vi "runtime execution.vi"() -> (0 "error out":errorcluster)   [LabVIEW 2013, in "shared memory module tests.lvlib"]
uses:
  shared memory module tests.lvlib
  module/execution/shared memory module runtime.lvclass
  module/execution/shared memory module runtime.lvclass/shared memory module runtime.ctl
  <vilib>/NI/Tag Bus/table/data polymorphs/write many/write Doubles.vi
  <vilib>/NI/Tag Bus/table/data polymorphs/write many/write I32s.vi
  <vilib>/NI/Tag Bus/table/data polymorphs/write many/write Booleans.vi
  module/execution/Read inputs.vi
  module/execution/Read outputs.vi
  <vilib>/NI/Tag Bus/table/data table.lvlib
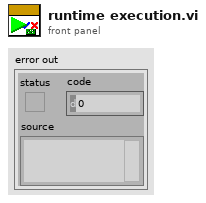
[diagram p1: front panel]
types:
  T1 = typedef "TBM channel.lvclass/data tables.ctl" = cluster{"input data":T2, "processing parameter":T2, "processing result":T2, "output data":T2}
  T2 = typedef "tag bus.lvlib/dictionary table pair.ctl" = cluster{"data dictionary":refnum<class "data dictionary.lvclass">, "data table":T3}
  T3 = typedef "tag bus.lvlib/data table.lvlib/data table.ctl" = cluster{"Double":dbl[], "Single":sgl[], "I64":i64[], "I32":i32[], "I16":i16[], "I8":i8[], "U64":u64[], "U32":u32[], "U16":u16[], "U8":u8[], "Boolean":bool[], "String":string[], "Array of Double":cluster{"DBL Array":dbl[]}[], "Array of Single":cluster{"SGL Array":sgl[]}[], "Array of I64":cluster{"I64 Array":i64[]}[], "Array of I32":cluster{"I32 Array":i32[]}[], "Array of I16":cluster{"I16 Array":i16[]}[], "Array of I8":cluster{"I8 Array":i8[]}[], "Array of U64":cluster{"U64 Array":u64[]}[], "Array of U32":cluster{"U32 Array":u32[]}[], "Array of U16":cluster{"U16 Array":u16[]}[], "Array of U8":cluster{"U8 Array":u8[]}[], "Array of Boolean":cluster{"Boolean Array":bool[]}[], "Array of String":cluster{"String Array":string[]}[]}
  T4 = typedef "current tag file io module runtime.lvclass/current tag file io configuration.ctl" = cluster{"refnum":refnum<file>, "name":string, "data type":T5, "number of tags":i32, "indices":cluster{"index":i32[]}, "data array":cluster{"data":dbl[]}, "file array":cluster{"data":dbl[]}}
  T5 = typedef "tag bus.lvlib/tag descriptor.lvclass/Data Type.ctl" = enum16{"Double", "Single", "I64", "I32", "I16", "I8", "U64", "U32", "U16", "U8", "Boolean", "String", "Array of Double", "Array of Single", "Array of I64", "Array of I32", "Array of I16", "Array of I8", "Array of U64", "Array of U32", "Array of U16", "Array of U8", "Array of Boolean", "Array of String"}
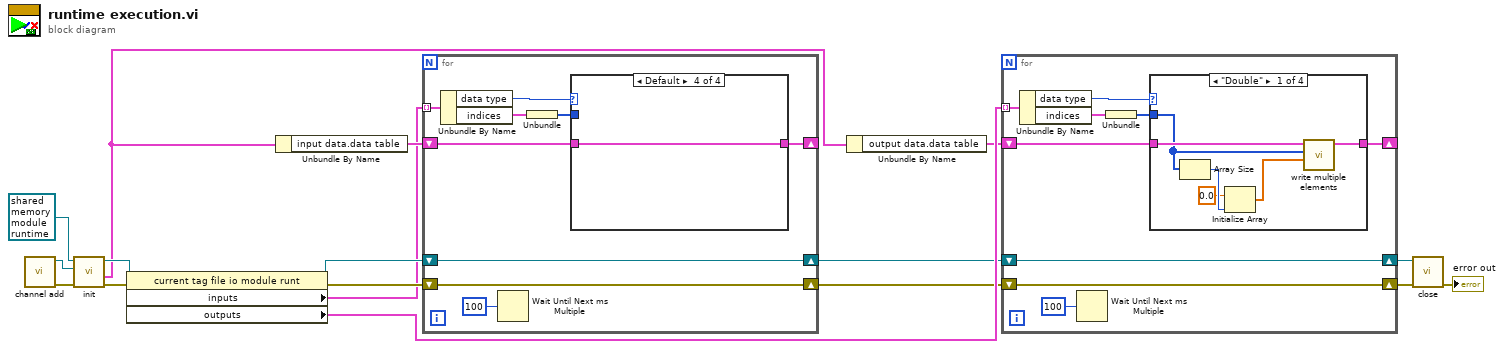
[diagram p0: block diagram]
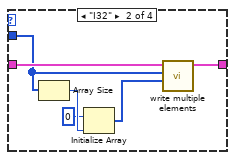
[diagram p2: hidden frame]
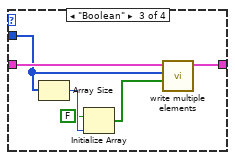
[diagram p3: hidden frame]
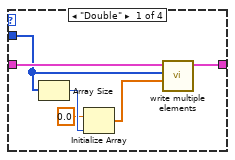
[diagram p5: hidden frame]
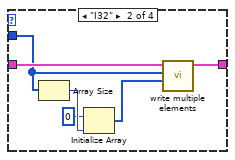
[diagram p6: hidden frame]
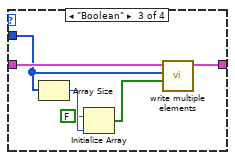
[diagram p7: hidden frame]
diagram:
  n1 = call "channel add.vi"() -> ("error out"=w15:errorcluster, "configuration out"=w17:refnum<class "shared memory module configuration.lvclass">)  [unwired: 7 in, 3 out]
  n2 = call-dynamic "init.vi"("error in"=w15, "TBM module configuration in"=w17, "file io module runtime in"=refnum<class "shared memory module runtime.lvclass"> refnum ("tag bus configurable plugin module")) -> ("error out"=w12:errorcluster, "data allocations"=w3:T1, "file io module runtime out"=w9:refnum<class "shared memory module runtime.lvclass">)  [unwired: 5 in, 1 out]
  n3 = property class="current tag file io module runt"(reference=w9, error in=w12) -> (reference out=w13:refnum<class "shared memory module runtime.lvclass">, error out=w11:errorcluster, "inputs"=w10:T4[], "outputs"=w8:T4[])
  n4 = Unbundle By Name(w3) -> ("input data.data table"=w14:T3)
  n5 = for {
    shift-right: [w18] -> w7
    shift-left: w13 -> [w18]
    shift-right: [w19] -> w6
    shift-left: w11 -> [w19]
    shift-right: [w20] -> _
    shift-left: w14 -> [w26]
    tunnel: w10 -> [w24] mode=indexing
    n6 = Unbundle By Name(w24) -> ("data type"=w22:T5, "indices"=w23:cluster{"index":i32[]})
    n7 = Wait Until Next ms Multiple(millisecond multiple=u32 100) -> ()  [unwired: 1 out]
    n8 = Unbundle(w23) -> ("index"=w21:i32[])
    n9 = case shown="Default" w22 {
      tunnel: w26 -> [w32 w38 w44 w45]
      tunnel: [w27 w33 w39 w45] -> w20
      tunnel: w21 -> [w31 w37 w43 _]
      frame "Double" {
        n10 = Array Size(array=w31) -> (size(s)=w30:i32)
        n11 = Initialize Array(0.0 ("element"), w30) -> (w28:dbl[])
        n12 = call-poly <vilib>:"write multiple elements.vi"("values"=w28, "indices"=w31, "data table in"=w32) -> ("data table out"=w27:T3)  [unwired: 8 in]
      }
      frame "I32" {
        n13 = Array Size(array=w37) -> (size(s)=w36:i32)
        n14 = Initialize Array(0 ("element"), w36) -> (w34:i32[])
        n15 = call-poly <vilib>:"write multiple elements.vi"("values"=w34, "indices"=w37, "data table in"=w38) -> ("data table out"=w33:T3)  [unwired: 8 in]
      }
      frame "Boolean" {
        n16 = Array Size(array=w43) -> (size(s)=w42:i32)
        n17 = Initialize Array(FALSE, w42) -> (w40:bool[])
        n18 = call-poly <vilib>:"write multiple elements.vi"("values"=w40, "indices"=w43, "data table in"=w44) -> ("data table out"=w39:T3)  [unwired: 8 in]
      }
      frame Default {
      }
    }
  }
  n19 = Unbundle By Name(w3) -> ("output data.data table"=w2:T3)
  n20 = for {
    shift-right: [w48] -> w5
    shift-left: w7 -> [w48]
    shift-right: [w47] -> w4
    shift-left: w6 -> [w47]
    shift-right: [w46] -> _
    shift-left: w2 -> [w54]
    tunnel: w8 -> [w52] mode=indexing
    n21 = Unbundle By Name(w52) -> ("data type"=w50:T5, "indices"=w51:cluster{"index":i32[]})
    n22 = Wait Until Next ms Multiple(millisecond multiple=u32 100) -> ()  [unwired: 1 out]
    n23 = Unbundle(w51) -> ("index"=w49:i32[])
    n24 = case shown="\"Double\"" w50 {
      tunnel: w54 -> [w60 w66 w72 w73]
      tunnel: [w55 w61 w67 w73] -> w46
      tunnel: w49 -> [w59 w65 w71 _]
      frame "Double" {
        n25 = Array Size(array=w59) -> (size(s)=w58:i32)
        n26 = Initialize Array(0.0 ("element"), w58) -> (w56:dbl[])
        n27 = call-poly <vilib>:"write multiple elements.vi"("values"=w56, "indices"=w59, "data table in"=w60) -> ("data table out"=w55:T3)  [unwired: 8 in]
      }
      frame "I32" {
        n28 = Array Size(array=w65) -> (size(s)=w64:i32)
        n29 = Initialize Array(0 ("element"), w64) -> (w62:i32[])
        n30 = call-poly <vilib>:"write multiple elements.vi"("values"=w62, "indices"=w65, "data table in"=w66) -> ("data table out"=w61:T3)  [unwired: 8 in]
      }
      frame "Boolean" {
        n31 = Array Size(array=w71) -> (size(s)=w70:i32)
        n32 = Initialize Array(FALSE, w70) -> (w68:bool[])
        n33 = call-poly <vilib>:"write multiple elements.vi"("values"=w68, "indices"=w71, "data table in"=w72) -> ("data table out"=w67:T3)  [unwired: 8 in]
      }
      frame Default {
      }
    }
  }
  n34 = call-dynamic "close.vi"("error in"=w4, "file io module runtime in"=w5) -> ("error out"=→"error out":errorcluster)  [unwired: 9 in]
